vi "02lectura_eeprom.vi"(3 "timeout ms":i32=500, 4 "puerto":i16=6340, 5 "Adress":string="192.168.1.6") -> (0 "error out":errorcluster, 1 "mapaeeprom":string, 2 "conn ID":refnum<k5>)   [LabVIEW 2010]
panel:
  out "pagina0":string
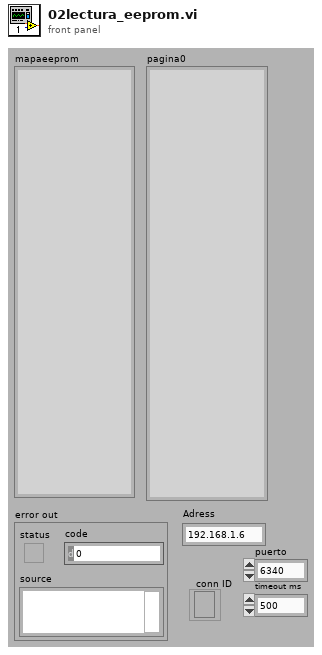
[diagram p1: front panel]
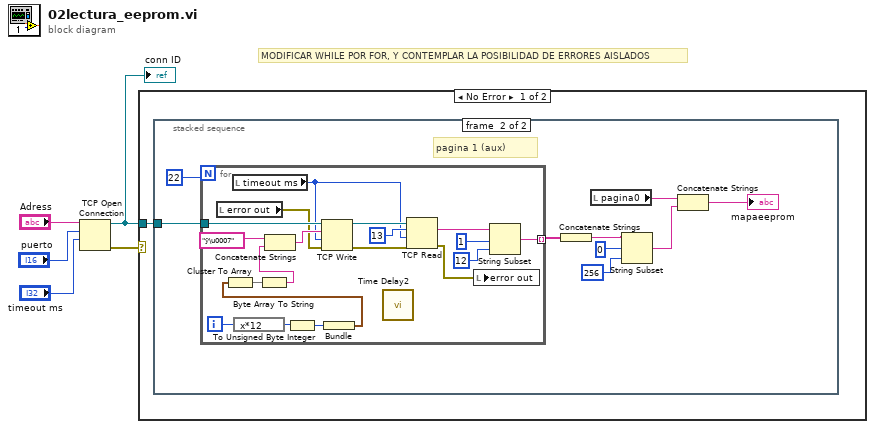
[diagram p0: block diagram]
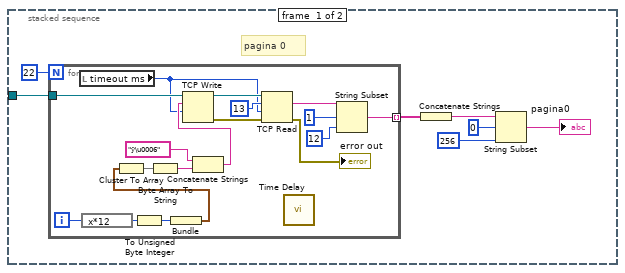
[diagram p2: hidden frame]
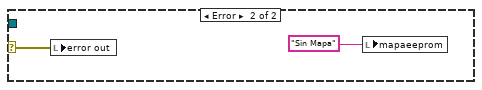
[diagram p3: hidden frame]
diagram:
  # "MODIFICAR WHILE POR FOR, Y CONTEMPLAR LA POSIBILIDAD DE ERRORES AISLADOS"
  n1 = TCP Open Connection(address="Adress", remote port or service name="puerto", timeout ms (60000)="timeout ms") -> (connection ID=w1:refnum<k5>, error out=w2:errorcluster)  [unwired: 1 in, 1 out]
  "conn ID" <- w1
  n2 = case shown="No Error" w2 {
    selector: w2 -> [_ w61]
    tunnel: w1 -> [w6 _]
    frame No Error {
      n3 = stacked-sequence {
        tunnel: w6 -> [w7 w35]
        frame #0 {
          # "pagina 0"
          n4 = for {
            N: 22 -> [_]
            tunnel: [w31] -> w12 mode=indexing
            tunnel: w7 -> [w27]
            i -> [w29]
            n5 = local read "timeout ms"() -> (w19:i32)
            n6 = expression code="x*12"(w29) -> (w18:i32)
            n7 = To Unsigned Byte Integer(number=w18) -> (unsigned 8bit integer=w17:u8)
            n8 = Bundle(w17) -> (w14:cluster{u8})  [unwired: 1 in]
            n9 = Cluster To Array(cluster=w14) -> (array=w15:u8[])
            n10 = Byte Array To String(unsigned byte array=w15) -> (string=w16:string)
            n11 = Concatenate Strings("ÿ\u0006" ("string to write"), w16) -> (w28:string)
            n12 = TCP Write(connection ID=w27, data in=w28, 9:w19) -> (connection ID out=w26:refnum<k5>, error out=w21:errorcluster)  [unwired: 1 in, 1 out]
            n13 = TCP Read(connection ID=w26, bytes to read=13, error in (no error)=w21, 9:w19) -> (data out=w23:string, error out=→"error out":errorcluster)  [unwired: 2 out]
            n14 = call "Time Delay"() -> ()  [unwired: 2 in, 10 out]
            n15 = String Subset(string=w23, offset (0)=1, length (rest)=12 ("length (rest)")) -> (substring=w31:string)
          }
          n16 = Concatenate Strings(w12) -> (w11:string)
          n17 = String Subset(string=w11, offset (0)=0, length (rest)=256 ("length (rest)")) -> (substring=→"pagina0":string)
        }
        frame #1 {
          # "pagina 1 (aux)"
          n18 = for {
            N: 22 -> [_]
            tunnel: [w59] -> w37 mode=indexing
            tunnel: w35 -> [w55]
            i -> [w56]
            n19 = local read "error out"() -> (w49:errorcluster)
            n20 = local read "timeout ms"() -> (w46:i32)
            n21 = expression code="x*12"(w56) -> (w45:i32)
            n22 = To Unsigned Byte Integer(number=w45) -> (unsigned 8bit integer=w44:u8)
            n23 = Bundle(w44) -> (w43:cluster{u8})  [unwired: 1 in]
            n24 = Cluster To Array(cluster=w43) -> (array=w42:u8[])
            n25 = Byte Array To String(unsigned byte array=w42) -> (string=w41:string)
            n26 = Concatenate Strings("ÿ\u0007" ("string to write"), w41) -> (w57:string)
            n27 = TCP Write(connection ID=w55, data in=w57, error in (no error)=w49, 9:w46) -> (connection ID out=w54:refnum<k5>, error out=w48:errorcluster)  [unwired: 1 out]
            n28 = call "Time Delay2"() -> ()  [unwired: 2 in, 10 out]
            n29 = TCP Read(connection ID=w54, bytes to read=u32 13 ("y"), error in (no error)=w48, 9:w46) -> (data out=w50:string, error out=w47:errorcluster)  [unwired: 2 out]
            n30 = local write "error out"(w47) -> ()
            n31 = String Subset(string=w50, offset (0)=1, length (rest)=12 ("length (rest)")) -> (substring=w59:string)
          }
          n32 = Concatenate Strings(w37) -> (w38:string)
          n33 = local read "pagina0"() -> (w34:string)
          n34 = String Subset(string=w38, offset (0)=0, length (rest)=256 ("length (rest)")) -> (substring=w32:string)
          n35 = Concatenate Strings(w34, w32) -> (→"mapaeeprom":string)
        }
      }
    }
    frame Error {
      n36 = local write "error out"(w61) -> ()
      n37 = local write "mapaeeprom"("Sin Mapa") -> ()
    }
  }
